vi "Create and Read DI.vi"(8 "error in":errorcluster, 10 "initial channel settings":T1[](array[typedef]), 11 "NI 9422 Test in":refnum<class "NI 9422 Test.lvclass">) -> (0 "error out":errorcluster, 2 "read channel settings":T1[](array[typedef]), 3 "NI 9422 Test out":refnum<class "NI 9422 Test.lvclass">)   [LabVIEW 2017, in "NI 9422 Test.lvclass"]
uses:
  NI 9422 Test.lvclass
  Scripting/Modules/Mode Classes/Controls/digital channel settings.ctl
  Scripting/Modules/NI 9422/NI 9422.lvclass
  Scripting/Scan Engine Scripting.lvlib
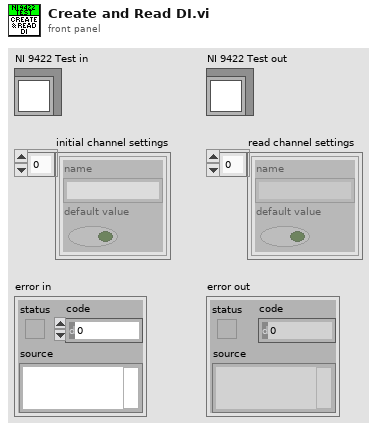
[diagram p1: front panel]
types:
  T1 = typedef "Scan Engine Scripting.lvlib/digital channel settings.ctl" = cluster{"name":string, "default value":bool}
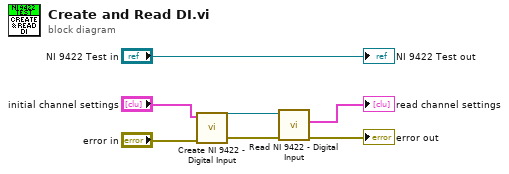
[diagram p0: block diagram]
diagram:
  n1 = call "Create NI 9422 - Digital Input.vi"("error in"="error in", "channel settings"="initial channel settings") -> ("error out"=w4:errorcluster, "NI 9422 out"=w5:refnum<class "NI 9422.lvclass">)  [unwired: 8 in]
  n2 = call "Read NI 9422 - Digital Input.vi"("error in"=w4, "NI 9422 in"=w5) -> ("error out"=→"error out":errorcluster, "channel settings"=→"read channel settings":T1[])  [unwired: 7 in, 1 out]
  "NI 9422 Test out" <- "NI 9422 Test in"
